vi "OAC.vi"(0 "System no.":i32=1 min=1 max=4 step=1, 2 "Axes to set":string[](array[string]), 3 "Acceleration values":dbl[](array[numeric]) format="%.6f", 4 "No.of digits":i16=4, 5 "error in":errorcluster, 6 "Without axis ID?":bool) -> (14 "Controller error":bool, 19 "error out":errorcluster)   [LabVIEW 2020]
doc: "Sets open-loop acceleration and checks for error. If Without axis ID? is TRUE, then Axes to set is ignored and first field of Acceleration values array is used for acceleration command. Number of digits is the number of digits after the decimal point in the acceleration value(s) that will be sent. Controller error is TRUE if selected system reports error code which is not 0.\n\nE-861, E-874: Without axis ID? = FALSE. Acceleration unit is steps/s²."
panel:
  # "Sets open-loop acceleration and checks for error.  If \"Without\naxis ID\" is TRUE, then \"Axes to set\" is ignored and first field of \nAcceleration values\" array is used for acceleration command."
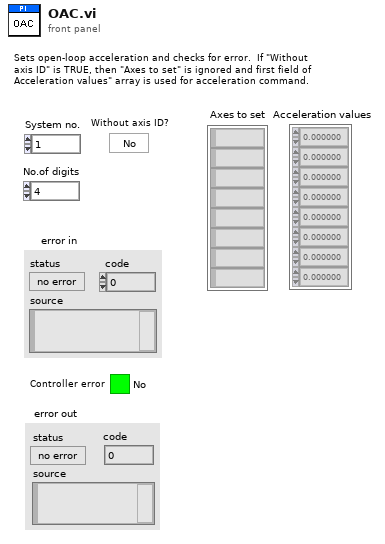
[diagram p1: front panel]
types:
  T1 = enum16{"Disable error check", "Force error check", "Use global settings"}
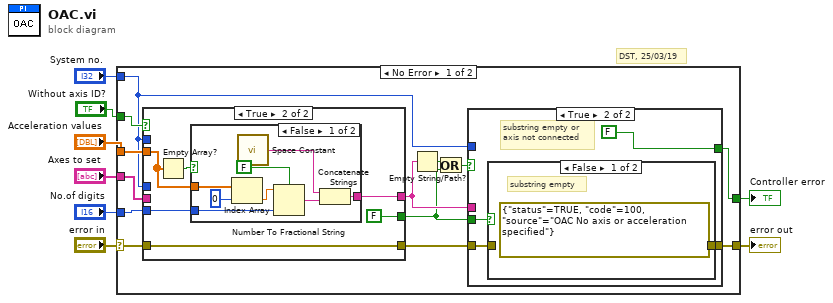
[diagram p0: block diagram]
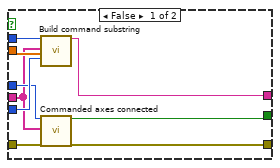
[diagram p2: hidden frame]
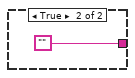
[diagram p3: hidden frame]
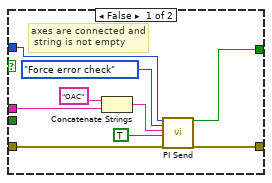
[diagram p4: hidden frame]
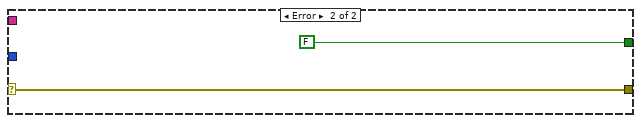
[diagram p6: hidden frame]
diagram:
  # "DST, 25/03/19"
  n1 = case shown="No Error" "error in" {
    selector: "error in" -> [w13 w61]
    tunnel: [w21 w61] -> w8
    tunnel: "Acceleration values" -> [w20 _]
    tunnel: "No.of digits" -> [w19 _]
    tunnel: "System no." -> [w15 _]
    tunnel: "Axes to set" -> [w17 _]
    tunnel: "Without axis ID?" -> [w16 _]
    tunnel: [w14 FALSE ("Controller error")] -> w2
    frame No Error {
      n2 = case shown="True" w16 {
        tunnel: [w30 w34] -> w10
        tunnel: w20 -> [w29 w33]
        tunnel: w19 -> [w28 w31]
        tunnel: w13 -> [w27 w36]
        tunnel: [w26 w36] -> w18
        tunnel: w15 -> [w25 _]
        tunnel: w17 -> [w24 _]
        tunnel: [w23 FALSE] -> w9
        tunnel: w15 -> [w22 _]
        frame False {
          n3 = call "Build command substring.vi"("System no."=w22, "Affected axes"=w24, "Parameters"=w29, "No. of digits"=w28) -> ("Command substring"=w30:string)  [unwired: 3 in, 12 out]
          n4 = call "Commanded axes connected.vi"("System no."=w25, "Commanded axes"=w24, "error in"=w27) -> ("Controller error"=w23:bool, "error out"=w26:errorcluster)  [unwired: 1 in, 14 out]
        }
        frame True {
          n5 = Empty Array?(array=w33) -> (empty?=w32:bool)
          n6 = case shown="False" w32 {
            tunnel: [w42 ""] -> w34
            tunnel: w33 -> [w41 _]
            tunnel: w31 -> [w39 _]
            frame False {
              n7 = Index Array(array=w41, index=0 ("Index")) -> (element=w40:dbl)
              n8 = call <vilib>:"Space Constant.vi"() -> ("String"=w43:string)
              n9 = Number To Fractional String(use system decimal point (T)=FALSE, number=w40, precision (6)=w39) -> (F-format string=w38:string)  [unwired: 1 out]
              n10 = Concatenate Strings(w43, w38) -> (w42:string)
            }
            frame True {
            }
          }
        }
      }
      n11 = Empty String/Path?(string/path=w10) -> (empty?=w11:bool)
      n12 = Or(x=w11, y=w9) -> (x .or. y?=w12:bool)
      n13 = case shown="True" w12 {
        tunnel: w10 -> [w53 _]
        tunnel: [w47 w58] -> w21
        tunnel: w18 -> [w50 w56]
        tunnel: w9 -> [_ w57]
        tunnel: w15 -> [w49 _]
        tunnel: [w46 FALSE ("Controller error")] -> w14
        frame False {
          # "axes are connected and\n string is not empty"
          n14 = Concatenate Strings("OAC", w53) -> (w51:string)
          n15 = call "PI Send.vi"("System no."=w49, "Error check settings"=T1."Force error check", "String to send"=w51, "Attach termination char.?"=TRUE ("Attach Linefeed?"), "error in"=w50) -> ("Controller error"=w46:bool, "error out"=w47:errorcluster)  [unwired: 1 in, 12 out]
        }
        frame True {
          # "substring empty or\naxis not connected"
          n16 = case shown="False" w57 {
            tunnel: [errorcluster {"status"=TRUE, "code"=100, "source"="OAC No axis or acceleration specified"} ("error out") w60] -> w58
            tunnel: w56 -> [_ w60]
            frame False {
              # "substring empty"
            }
            frame True {
              # "commanded axis\nnot connected"
            }
          }
        }
      }
    }
    frame Error {
    }
  }
  "error out" <- w8
  "Controller error" <- w2
